vi "Concatenate Status Text String.vi"(7 "Max Number of Messages to Display":i32=10, 9 "Severity":u8, 10 "New Status Message":string, 11 "Status Text":string) -> (3 "Output":string)   [LabVIEW 2014]
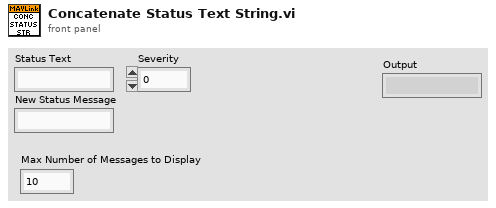
[diagram p1: front panel]
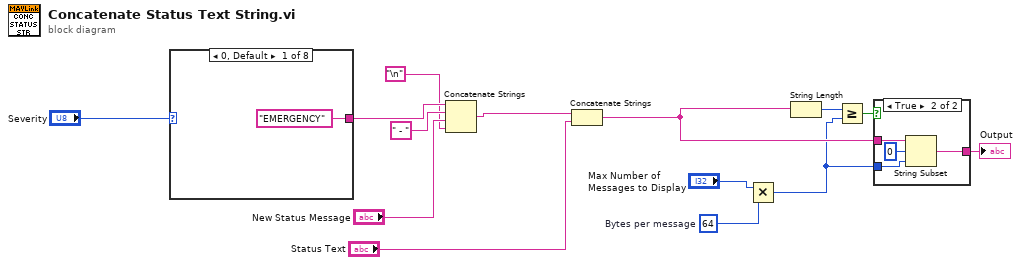
[diagram p0: block diagram]
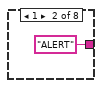
[diagram p2: hidden frame]
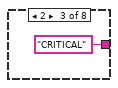
[diagram p3: hidden frame]
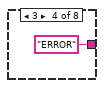
[diagram p4: hidden frame]
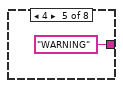
[diagram p5: hidden frame]
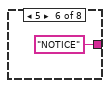
[diagram p6: hidden frame]
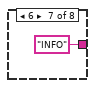
[diagram p7: hidden frame]
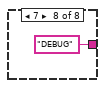
[diagram p8: hidden frame]
diagram:
  w3 = 64  # Bytes per message
  n1 = case shown="0, Default" "Severity" {
    tunnel: ["EMERGENCY" "ALERT" "CRITICAL" "ERROR" "WARNING" "NOTICE" "INFO" "DEBUG"] -> w10
    frame 0, Default {
    }
    frame 1 {
    }
    frame 2 {
    }
    frame 3 {
    }
    frame 4 {
    }
    frame 5 {
    }
    frame 6 {
    }
    frame 7 {
    }
  }
  n2 = Concatenate Strings(w10, " - " ("string"), "New Status Message", "\n") -> (w7:string)
  n3 = Concatenate Strings(w7, "Status Text") -> (w5:string)
  n4 = Multiply(x="Max Number of Messages to Display", y=w3) -> (x*y=w2:i32)
  n5 = String Length(string=w5) -> (length=w13:i32)
  n6 = Greater Or Equal?(x=w13, y=w2) -> (x >= y?=w14:bool)
  n7 = case shown="True" w14 {
    tunnel: [w23 w27] -> w12
    tunnel: w5 -> [w23 w26]
    tunnel: w2 -> [_ w24]
    frame False {
    }
    frame True {
      n8 = String Subset(string=w26, offset (0)=0, length (rest)=w24) -> (substring=w27:string)
    }
  }
  "Output" <- w12
